vi "Remove_TrainingExamples.vi"(9 "rooth path":path=path "C:/smasoft/system", 10 "number":string, 11 "package":string) -> ()   [LabVIEW 2019]
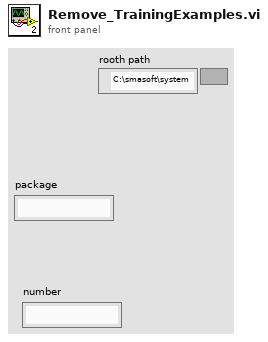
[diagram p1: front panel]
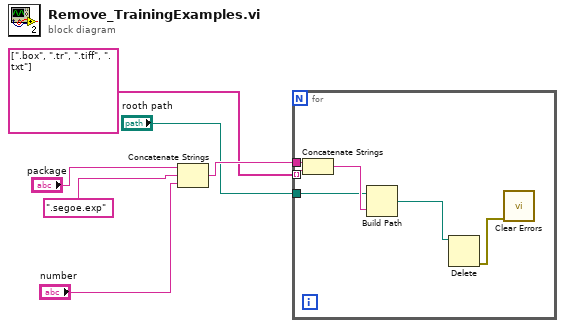
[diagram p0: block diagram]
diagram:
  n1 = Concatenate Strings("package", ".segoe.exp" ("string"), "number") -> (w3:string)
  n2 = for {
    tunnel: w3 -> [w12]
    tunnel: string[] [".box", ".tr", ".tiff", ".txt"] ("string") -> [w11] mode=indexing
    tunnel: "rooth path" -> [w9]
    n3 = Concatenate Strings(w12, w11) -> (w10:string)
    n4 = Build Path(base path=w9, name or relative path=w10) -> (appended path=w8:path)
    n5 = Delete(path (use dialog)=w8) -> (error out=w7:errorcluster)  [unwired: 4 in, 2 out]
    n6 = call <vilib>:"Clear Errors.vi"("error in (no error)"=w7) -> ()  [unwired: 5 in, 2 out]
  }
